vi "dialog.one_button_lua.vi"(5 "LuaVIEW reference":T1) -> (15 "error out":errorcluster)   [LabVIEW 2012]
doc: "Display a one-button dialog with a message. Returns when the button is clicked, the dialog window is closed or either the Return or Escape keys are pressed.\n\nThe shown dialog is functionally identical to the standard LabVIEW \"One Button Dialog\". The standard dialog is not used because, at least up to LabVIEW version 7.1, it has the nasty property that it blocks the user interface thread while open. The UI thread is required not just for display updates but also for VI loading and instantiation. Thus, using the standard \"One Button Dialog\" might prevent essential background tasks from doing their job.\n\nBeware that the dialog pops up on the machine running Lua, which may not be the same as the machine being operated by the user in case of a client-server setup.\nParameters:\nstr:message. message to display in the dialog box.\nstr:button, text to display on the button, e.g. \"OK\"."
uses:
  typedefs/t_LuaVIEW Reference.ctl
  subvis/private/LuaVIEW Pull (string).vi
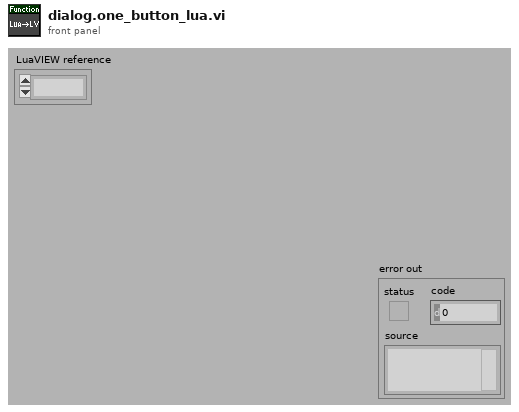
[diagram p1: front panel]
types:
  T1 = typedef "t_LuaVIEW Reference.ctl" = refnum<k1>
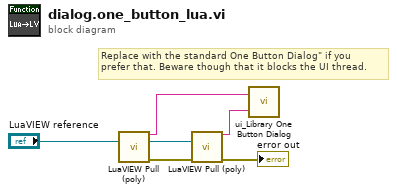
[diagram p0: block diagram]
diagram:
  # "Replace with the standard One Button Dialog\" if you\nprefer that. Beware though that it blocks the UI thread."
  n1 = call-poly "LuaVIEW Pull (poly).vi"("LuaVIEW reference in"="LuaVIEW reference") -> ("string"=w4:string, "LuaVIEW reference out"=w6:T1, "error out"=w1:errorcluster)  [unwired: 12 in]
  n2 = call-poly "LuaVIEW Pull (poly).vi"("LuaVIEW reference in"=w6, "error in (no error)"=w1) -> ("string"=w3:string, "error out"=→"error out":errorcluster)  [unwired: 11 in, 1 out]
  n3 = call "ui_Library One Button Dialog.vi"("button name (\"OK\")"=w3, "message"=w4) -> ()  [unwired: 1 out]
